vi "Mean and Standard Deviation.vi"(11 "Data Sets in":refnum<class "JSON Object.lvclass">[](array[class])) -> (3 "Means and Standard Deviations":refnum<class "JSON Value.lvclass">)   [LabVIEW 2020, in "Library Commun.lvlib" / "JSON Statistics.lvclass"]
doc: "Performs statistics on an array of JSON Data Sets. Each numeric in the JSON will have its mean calculated. If the numeric is varying, a Standard Deviation will also be calculated and added as an additional item, of the same name, but with \"(SD)\" added. Non numeric items are included in the output."
uses:
  JSON Statistics.lvclass
  JSON Value/JSON Value.lvclass
  JSON Object/JSON Object.lvclass
  C:/Users/ngarcin/OneDrive - Altyor/Standard TB/Class/JSON API/JSON Value/JSON Value.lvclass
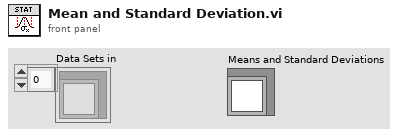
[diagram p1: front panel]
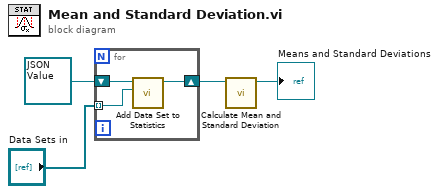
[diagram p0: block diagram]
diagram:
  n1 = for {
    tunnel: "Data Sets in" -> [w7] mode=indexing
    shift-right: [w5] -> w2
    shift-left: refnum<class "JSON Value.lvclass"> refnum ("JSON Value In") -> [w6]
    n2 = call "Add Data Set to Statistics.vi"("JSON Data Set"=w7, "Statistics in"=w6) -> ("Statistics"=w5:refnum<class "JSON Value.lvclass">)  [unwired: 9 in]
  }
  n3 = call "Calculate Mean and Standard Deviation.vi"("Statistics in"=w2) -> ("Mean and Standard Deviation(SD)"=→"Means and Standard Deviations":refnum<class "JSON Value.lvclass">)  [unwired: 10 in]
